vi "Set SPI PHY Configuration for SPI Transaction.vi"(7 "Chip Select":u8, 8 "error in":errorcluster, 9 "Set?":bool=TRUE, 10 "SPI PHY Settings":T1={"Divide Value"=20, "Transfer Length (bits)"=32, "CS Asserted Polarity"=FALSE, "Clock Polarity (CPOL)"=FALSE, "Clock Phase (CPHA)"=FALSE, "Lengthen MISO Setup"=FALSE, "Direction Change Bit"=0, "MOSI Starts as Output"=FALSE, "Tristatable MOSI"=FALSE} {"Direction Change Bit" max=64 step=1; "Transfer Length (bits)" min=1 max=64 step=1}, 11 "Private Data In":T2={"DLU To SPI Engine Data FIFO"="DLU To SPI Engine Data", "SPI Engine to DLU Data FIFO"="SPI Engine to DLU Data", "Data to SPI Engine (Cache) Register"="Data to SPI Engine (Cache)", "SPI PHY Settings to SPI Engine (Cahche) Register"="SPI PHY Settings to SPI Engine (Cache)"}) -> (0 "error out":errorcluster, 3 "Private Data Out":T2={"DLU To SPI Engine Data FIFO"="DLU To SPI Engine Data", "SPI Engine to DLU Data FIFO"="SPI Engine to DLU Data", "Data to SPI Engine (Cache) Register"="Data to SPI Engine (Cache)", "SPI PHY Settings to SPI Engine (Cahche) Register"="SPI PHY Settings to SPI Engine (Cache)"})   [LabVIEW 2014]
doc: "This VI Configures SPI Settings for the required channel (using Chip Select ID) on SPI bus.s"
uses:
  Controls/Internal Data (SPI API).ctl
  user.lib/_NI SPI IP/FPGA/Controllers/Public/Transfer Settings.ctl
  <vilib>/Utility/error.llb/Clear Errors.vi
  <vilib>/rvi/Emulation/niFpgaSctlEmulationGetInTimedLoop.vi
  <vilib>/rvi/DataTransferAndStorage/Container/Common/niFpgaContainerExecOnDevCompGetState.vi
  <vilib>/rvi/Emulation/niFpgaEmulationIsFPGAContextNoSignature.vi
  <vilib>/rvi/DataTransferAndStorage/Container/Common/niFpgaContainerGetUniqueNameForEmu.vi
  <vilib>/rvi/Memory/Memory_Emulation/niFpgaMemoryEmulationCacheClearOnFirstRun.vi
  <vilib>/rvi/Memory/Memory_Emulation/nirvimemoryEmulationManagerCache_MakeExclusive.vi
  <vilib>/rvi/Memory/Memory_Emulation/niFpgaMemoryEmulationValidateCache.vi
  <vilib>/rvi/Memory/Memory_Emulation/nirvimemoryEmulationManagerCache_InsertValue.vi
  <vilib>/rvi/Memory/Memory_Emulation/nirvimemoryEmulationManagerCache_ReleaseExclusive.vi
  <vilib>/rvi/Memory/Memory_Emulation/nirvimemoryEmulationManagerCache_GetValue.vi
  <vilib>/rvi/Memory/Memory_Emulation/nirvimemoryEmulationManagerCache_SetValue.vi
  <vilib>/rvi/Emulation/niFpgaProcessEmulError.vi
  <vilib>/rvi/DataTransferAndStorage/Container/XNode/niFpgaContainer.xnode
  <vilib>/rvi/DataTransferAndStorage/Register/Emulation/niFpgaRegisterEmulationRefIn.vi
  user.lib/_NI SPI IP/FPGA/Controllers/NI SPI IP (FPGA).lvlib
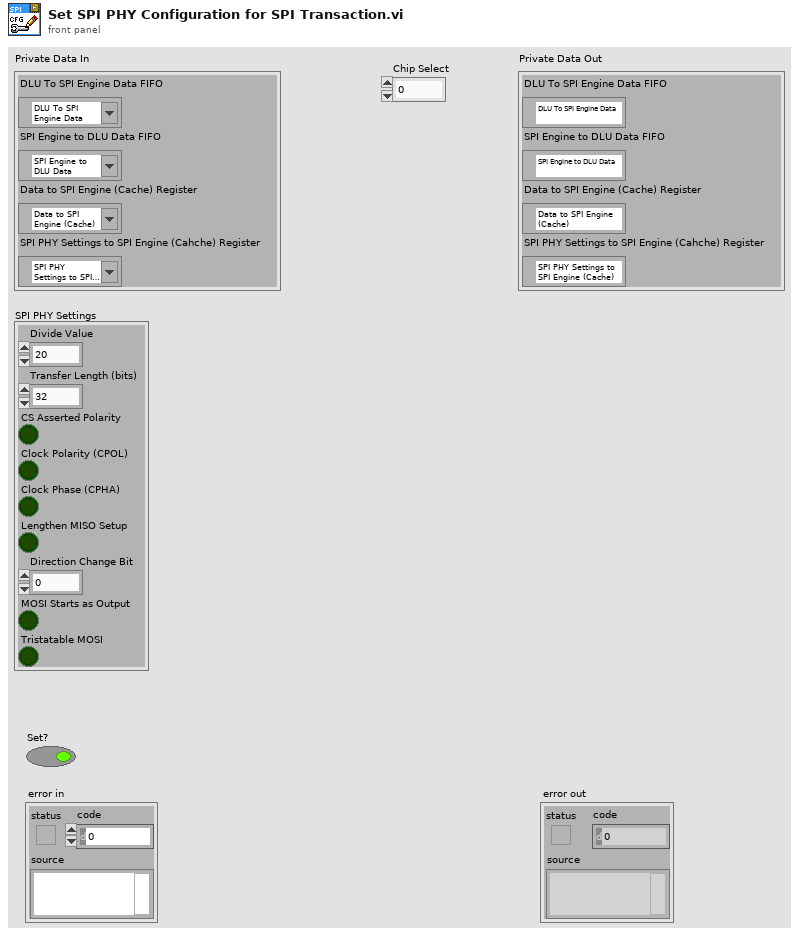
[diagram p1: front panel]
types:
  T1 = typedef "NI SPI IP (FPGA).lvlib/Transfer Settings.ctl" = cluster{"Divide Value":u8, "Transfer Length (bits)":u8, "CS Asserted Polarity":bool, "Clock Polarity (CPOL)":bool, "Clock Phase (CPHA)":bool, "Lengthen MISO Setup":bool, "Direction Change Bit":u8, "MOSI Starts as Output":bool, "Tristatable MOSI":bool}
  T2 = typedef "Internal Data (SPI API).ctl" = cluster{"DLU To SPI Engine Data FIFO":refnum<k21>, "SPI Engine to DLU Data FIFO":refnum<k21>, "Data to SPI Engine (Cache) Register":refnum<k21>, "SPI PHY Settings to SPI Engine (Cahche) Register":refnum<k21>}
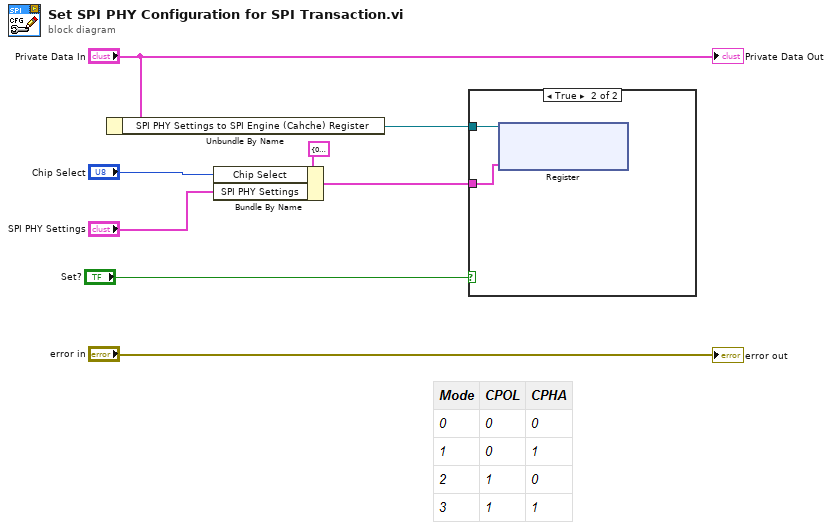
[diagram p0: block diagram]
diagram:
  n1 = Unbundle By Name("Private Data In") -> ("SPI PHY Settings to SPI Engine (Cahche) Register"=w3:refnum<k21>)
  n2 = Bundle By Name(cluster=cluster{"Chip Select":u8, "SPI PHY Settings":T1} {"Chip Select"=0, "SPI PHY Settings"={"Divide Value"=0, "Transfer Length (bits)"=0, "CS Asserted Polarity"=FALSE, "Clock Polarity (CPOL)"=FALSE, "Clock Phase (CPHA)"=FALSE, "Lengthen MISO Setup"=FALSE, "Direction Change Bit"=0, "MOSI Starts as Output"=FALSE, "Tristatable MOSI"=FALSE}} ("output cluster"), "Chip Select"="Chip Select", "SPI PHY Settings"="SPI PHY Settings") -> (w2:cluster{"Chip Select":u8, "SPI PHY Settings":T1})
  n3 = case shown="True" "Set?" {
    tunnel: w3 -> [_ w10]
    tunnel: w2 -> [_ w9]
    frame False {
    }
    frame True {
      n4 = xnode "Register"("Data"=w9, "Register In"=w10) -> ()  [unwired: 1 out]
    }
  }
  "Private Data Out" <- "Private Data In"
  "error out" <- "error in"
